vi "addField.vi"(6 "col":i32, 9 "row":i32, 10 "value":i32, 11 "BingoBoard in":refnum<class "BingoBoard.lvclass">) -> (3 "BingoBoard out":refnum<class "BingoBoard.lvclass">)   [LabVIEW 2017, in "BingoBoard.lvclass"]
uses:
  BingoBoard.lvclass
  BingoBoard.lvclass/BingoBoard.ctl
  BoardField/BoardField.lvclass
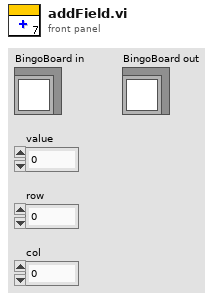
[diagram p1: front panel]
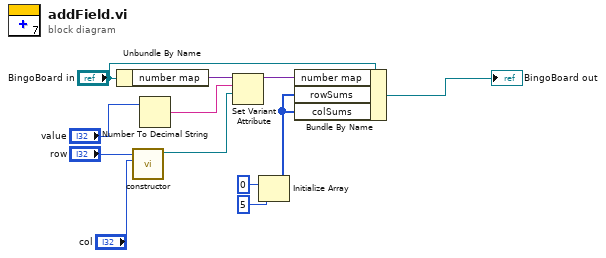
[diagram p0: block diagram]
diagram:
  n1 = Unbundle By Name("BingoBoard in") -> ("number map"=w6:variant)
  n2 = call "constructor.vi"("col"="col", "row"="row") -> ("field"=w9:refnum<class "BoardField.lvclass">)  [unwired: 9 in]
  n3 = Number To Decimal String(number="value") -> (decimal integer string=w8:string)  [unwired: 1 in]
  n4 = Set Variant Attribute(Variant=w6, name=w8, value=w9) -> (Variant out=w11:variant)  [unwired: 1 in, 2 out]
  n5 = Initialize Array(0 ("element"), 5 ("dimension size")) -> (w1:i32[])
  n6 = Bundle By Name(cluster="BingoBoard in", "number map"=w11, "rowSums"=w1, "colSums"=w1) -> (→"BingoBoard out":refnum<class "BingoBoard.lvclass">)
